vi "PLL_PID.vi"(9 "REF []":waveform(dbl), 10 "AO []":waveform(dbl)) -> (1 "phase output":dbl, 2 "frequency output":dbl)   [LabVIEW 2016, in "LockinDAQ.lvclass"]
doc: "Please ensure that at least one period is generated or else the measurement VIs do not work properly."
uses:
  LockinDAQ.lvclass
  <vilib>/measure/matone.llb/Extract Single Tone Information 1 Chan.vi
  <vilib>/addons/control/pid/pid.llb/PID (DBL).vi
  <vilib>/Analysis/NI_AALPro.lvlib
  <vilib>/measure/NI_MAPro.lvlib
  <vilib>/addons/control/pid/NI_PID_pid.lvlib
panel:
  out "process frequency":dbl format="%.2p"
  out "detected frequency":dbl format="%.2p"
  in  "PID_Phase":T1={"proportional gain (Kc)"=0.1, "integral time (Ti, min)"=0.0008, "derivative time (Td, min)"=0.0} {"derivative time (Td, min)" format="%.3f"; "integral time (Ti, min)" items=["Take a Coffee"=0.1, "Yawning"=0.01, "Take a Deep Breath"=0.001, "Normal"=0.0008, "A Little Bit Fast"=0.0001, "Fast"=1e-05, "Too Fast"=1e-06]; "proportional gain (Kc)" format="%.3f"}
  out "Current Frequency [Hz]":dbl=10.000000000000004 format="%.2f"
  in  "PID_Frequency":T1={"proportional gain (Kc)"=0.9, "integral time (Ti, min)"=0.0008, "derivative time (Td, min)"=0.0} {"derivative time (Td, min)" format="%.3f"; "integral time (Ti, min)" items=["Take a Coffee"=0.1, "Yawning"=0.01, "Take a Deep Breath"=0.001, "Normal"=0.0008, "A Little Bit Fast"=0.0001, "Fast"=1e-05, "Too Fast"=1e-06]; "proportional gain (Kc)" format="%.3f"}
  out "Waveform Graph":waveform(dbl)[](graph)=[{"t0"=timestamp(0 s since 1904-01-01), "dt"=0.001, "Y"=array[1000 elements]}, {"t0"=timestamp(0 s since 1904-01-01), "dt"=0.001, "Y"=array[1000 elements]}]
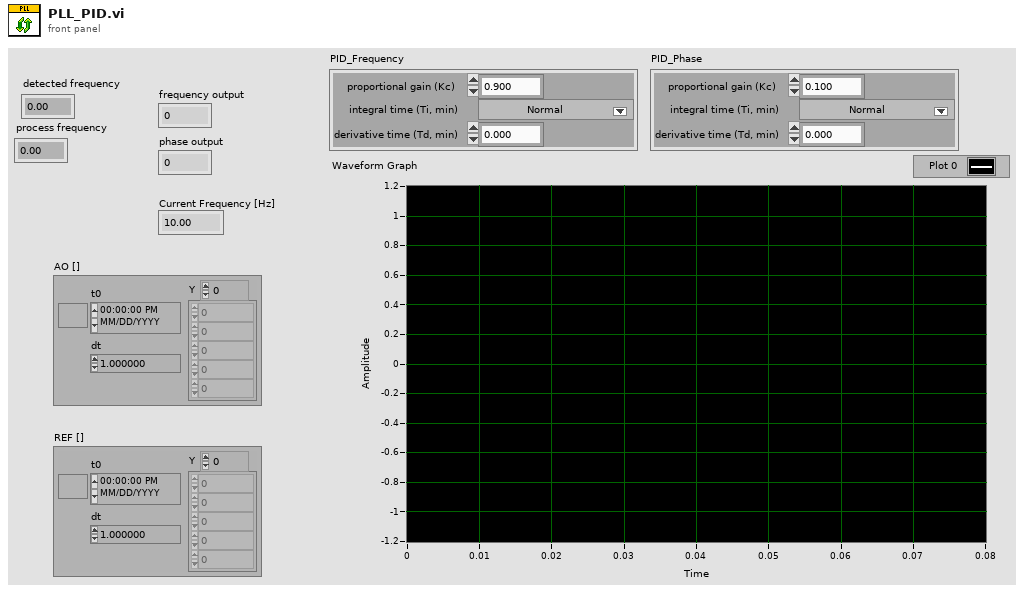
[diagram p1: front panel]
types:
  T1 = cluster{"proportional gain (Kc)":dbl, "integral time (Ti, min)":dbl, "derivative time (Td, min)":dbl}
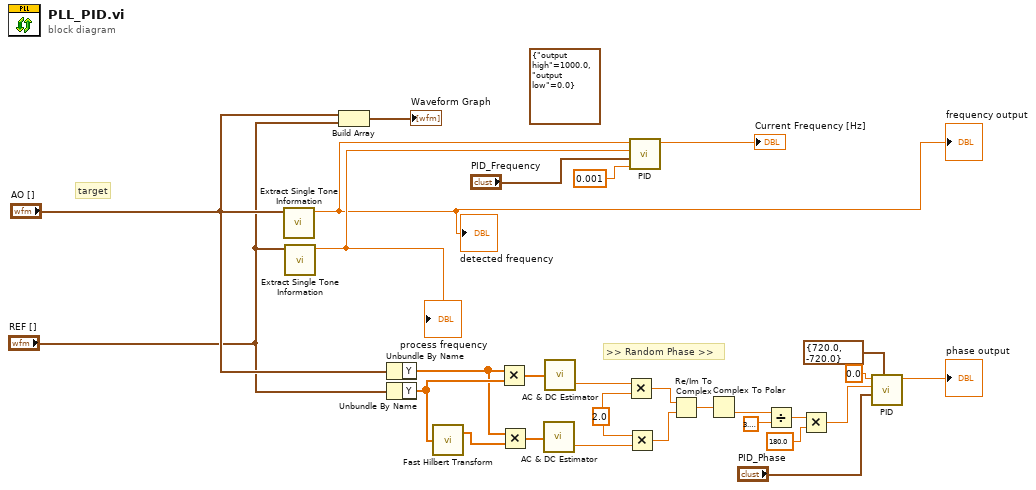
[diagram p0: block diagram]
diagram:
  (unwired) cluster{"output high":dbl, "output low":dbl} {"output high"=1000.0, "output low"=0.0} ("output range")
  w12 = 2.0 ("x")
  # "target"
  # ">> Random Phase >>"
  n1 = call-poly <vilib>:"Extract Single Tone Information.vi"("time signal in"="AO []") -> ("detected frequency"=w1:dbl)  [unwired: 5 in, 5 out]
  "frequency output" <- w1
  "detected frequency" <- w1
  n2 = call-poly <vilib>:"Extract Single Tone Information.vi"("time signal in"="REF []") -> ("detected frequency"=w10:dbl)  [unwired: 5 in, 5 out]
  "process frequency" <- w10
  n3 = Build Array("AO []", "REF []") -> (→"Waveform Graph":waveform(dbl)[])
  n4 = Unbundle By Name("AO []") -> ("Y"=w24:dbl[])
  n5 = Unbundle By Name("REF []") -> ("Y"=w26:dbl[])
  n6 = call <vilib>:"Fast Hilbert Transform.vi"("X"=w26) -> ("Hilbert{X}"=w25:dbl[])  [unwired: 1 out]
  n7 = Multiply(x=w24, y=w26) -> (x*y=w23:dbl[])
  n8 = Multiply(x=w24, y=w25) -> (x*y=w22:dbl[])
  n9 = call <vilib>:"AC & DC Estimator.vi"("Signal (V)"=w22) -> ("DC estimate (V)"=w21:dbl)  [unwired: 1 out]
  n10 = call <vilib>:"AC & DC Estimator.vi"("Signal (V)"=w23) -> ("DC estimate (V)"=w13:dbl)  [unwired: 1 out]
  n11 = Multiply(x=w13, y=w12) -> (x*y=w15:dbl)
  n12 = Multiply(x=w12, y=w21) -> (x*y=w14:dbl)
  n13 = call-poly <vilib>:"PID.vi"("dt (s)"=0.001, "PID gains"="PID_Frequency", "process variable"=w10, "setpoint"=w1) -> ("output"=→"Current Frequency [Hz]":dbl)  [unwired: 6 in, 1 out]
  n14 = Re/Im To Complex(1:w14, 2:w15) -> (0:w16:cdb)
  n15 = Complex To Polar(r * e^(i*theta)=w16) -> (theta=w17:dbl)  [unwired: 1 out]
  n16 = Divide(x=w17, y=3.141592653589793) -> (x/y=w19:dbl)
  n17 = Multiply(x=w19, y=180.0) -> (x*y=w7:dbl)
  n18 = call-poly <vilib>:"PID.vi"("output range"=cluster{"output high":dbl, "output low":dbl} {"output high"=720.0, "output low"=-720.0}, "PID gains"="PID_Phase", "process variable"=w7, "setpoint"=0.0) -> ("output"=→"phase output":dbl)  [unwired: 6 in, 1 out]
